vi "RoboArm_v5.vi"() -> ()   [LabVIEW 2013]
panel:
  out "S2":i32
  out "S:":i32
  out "F: 2":i32
  out "A: 2":i32
  in  "Y mm":dbl(knob) scale=150.0..300.0
  in  "Z mm":dbl(knob) scale=-100.0..300.0
  out "F:":i32
  out "A:":i32
  out "a1 =":dbl
  out "a2 =":dbl
  out "a3 =":dbl
  out "OF(B5) =":dbl
  out "OA(B1) =":dbl
  out "XY Graph 2":cluster{dbl[], dbl[]}(graph)
  in  "stop":bool
  # "Coordinates of joints:"
  # "Z"
  # "Y"
  # "Distances for joints:"
  # "Angel for every joint:"
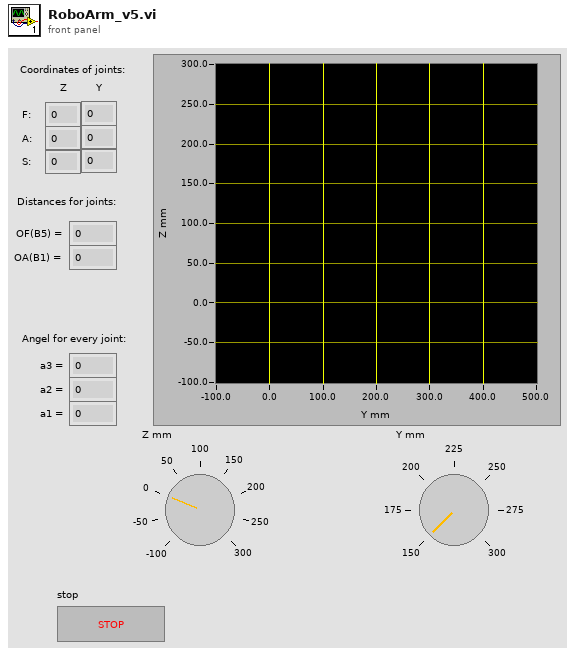
[diagram p1: front panel]
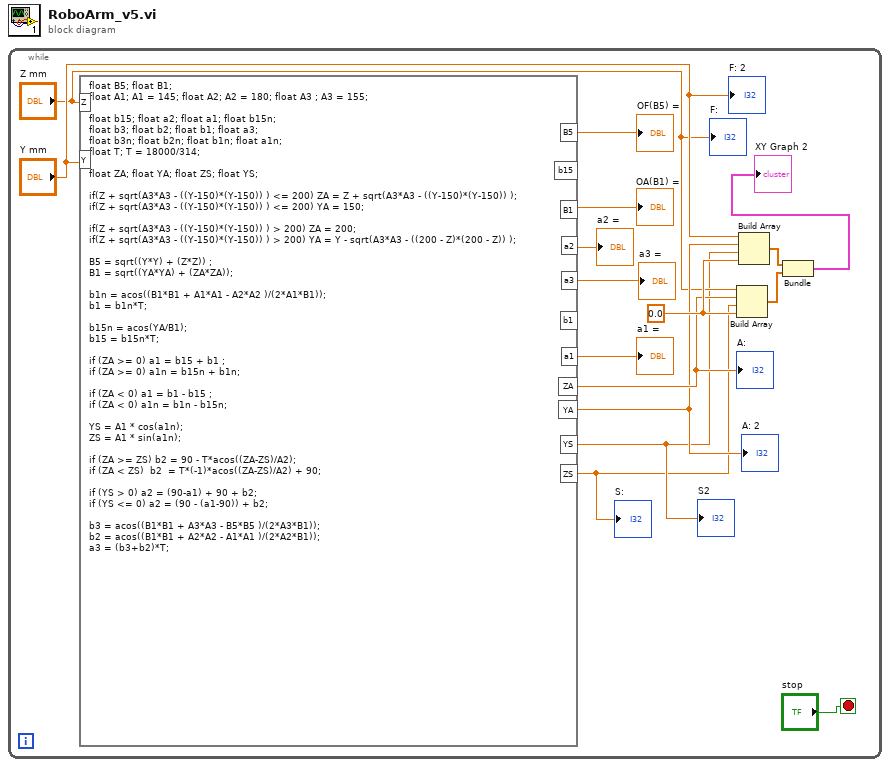
[diagram p0: block diagram]
diagram:
  n1 = while {
    stop <- "stop" stop-if-true
    w10 = 0.0 ("element")
    n2 = formula code="float B5; float B1;\nfloat A1; A1 = 145; float A2; A2 = 180; float A3 ; A3 = 155;\n\nfloat b15; float a2; float a1; float b15n;\nfloat b3; float b2; float b1; float a3;\nfloat b3n; float b2n; float b1n; float a1n;\nfloat T; T = 18000/314;\n\nfloat ZA; float YA; float ZS; float YS;\n\nif(Z + sqrt(A3*A3 - ((Y-150)*(Y-150)) ) <= 200) ZA = Z + sqrt(A3*A3 - ((Y-150)*(Y-150)) );\nif(Z + sqrt(A3*A3 - ((Y-150)*(Y-150)) ) <= 200) YA = 150; \n\nif(Z + sqrt(A3*A3 - ((Y-150)*(Y-150)) ) > 200) ZA = 200; \nif(Z + sqrt(A3*A3 - ((Y-150)*(Y-150)) ) > 200) YA = Y - sqrt(A3*A3 - ((200 - Z)*(200 - Z)) );\n\nB5 = sqrt((Y*Y) + (Z*Z)) ;\nB1 = sqrt((YA*YA) + (ZA*ZA));\n\nb1n = acos((B1*B1 + A1*A1 - A2*A2 )/(2*A1*B1));\nb1 = b1n*T;\n\nb15n = acos(YA/B1);\nb15 = b15n*T;\n\nif (ZA >= 0) a1 = b15 + b1 ;\nif (ZA >= 0) a1n = b15n + b1n;\n\nif (ZA < 0) a1 = b1 - b15 ;\nif (ZA < 0) a1n = b1n - b15n;\n\nYS = A1 * cos(a1n);\nZS = A1 * sin(a1n);\n\nif (ZA >= ZS) b2 = 90 - T*acos((ZA-ZS)/A2);\nif (ZA < ZS)  b2  = T*(-1)*acos((ZA-ZS)/A2) + 90;\n \nif (YS > 0) a2 = (90-a1) + 90 + b2;\nif (YS <= 0) a2 = (90 - (a1-90)) + b2;\n\nb3 = acos((B1*B1 + A3*A3 - B5*B5 )/(2*A3*B1));\nb2 = acos((B1*B1 + A2*A2 - A1*A1 )/(2*A2*B1));\na3 = (b3+b2)*T;"("Z"="Z mm", "Y"="Y mm") -> ("B5"=→"OF(B5) =":dbl, "B1"=→"OA(B1) =":dbl, "a1"=→"a1 =":dbl, "ZA"=w8:dbl, "YA"=w7:dbl, "YS"=w2:dbl, "ZS"=w1:dbl, "a2"=→"a2 =":dbl, "a3"=→"a3 =":dbl)  [unwired: 2 out]
    "A:" <- w8
    "A: 2" <- w7
    "S:" <- w1
    "S2" <- w2
    n3 = Build Array("Z mm", w8, w1, w10) -> (w11:dbl[])
    n4 = Build Array("Y mm", w7, w2, w10) -> (w13:dbl[])
    n5 = Bundle(w13, w11) -> (→"XY Graph 2":cluster{dbl[], dbl[]})  [unwired: 1 in]
    "F:" <- "Z mm"
    "F: 2" <- "Y mm"
  }
